vi "LED!!!!!s.vi"() -> ()   [LabVIEW 2020]
uses:
  LED GLOBALS!!!.vi
  LED-Global-string-length.vi
panel:
  out "Boolean":bool
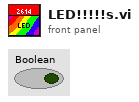
[diagram p1: front panel]
types:
  T1 = typedef "LED_Control_States.ctl" = enum16{"Config-Stripes", "swapperlines", "Rand", "Solid", "Flash-S", "Gradyent", "Move-Stripes", "Org-Rand", "Move-Point-Tail", "Flames", "Fade", "Alt-Colors"}
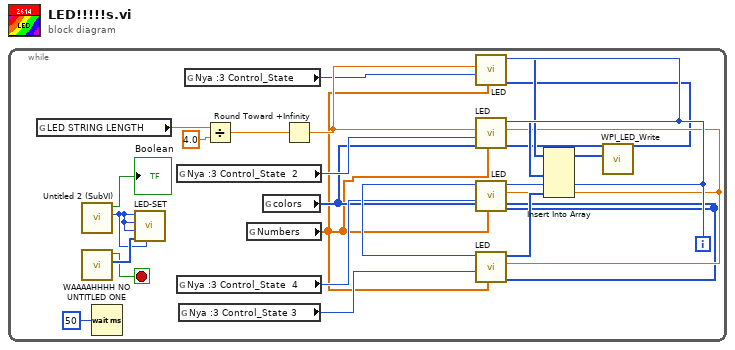
[diagram p0: block diagram]
diagram:
  n1 = while {
    i -> [w20]
    stop <- w3 stop-if-true
    n2 = global read "LED-Global-string-length.vi" "LED STRING LENGTH"() -> (w8:dbl)
    n3 = call "Untitled 2 (SubVI).vi"() -> ("Control_State"=w2:T1, "Boolean"=→"Boolean":bool)  [unwired: 10 in]
    n4 = call "WAAAAHHHH NO UNTITLED ONE.vi"() -> ("Array"=w4:u32[], "Boolean"=w3:bool)  [unwired: 10 in]
    n5 = Wait (ms)(milliseconds to wait=u32 50) -> ()  [unwired: 1 out]
    n6 = call "LED-SET.vi"("Control_State"=w2, "colors"=w4, "Control_State 2"=w2, "Control_State 3"=w2, "Control_State 4"=w2) -> ()  [unwired: 7 in]
    n7 = global read "LED GLOBALS!!!.vi" "Nya :3 Control_State  2"() -> (w11:T1)
    n8 = global read "LED GLOBALS!!!.vi" "Nya :3 Control_State  4"() -> (w9:T1)
    n9 = global read "LED GLOBALS!!!.vi" "Nya :3 Control_State 3"() -> (w10:T1)
    n10 = global read "LED GLOBALS!!!.vi" "Nya :3 Control_State"() -> (w12:T1)
    n11 = Divide(x=w8, y=4.0) -> (x/y=w15:dbl)
    n12 = global read "LED GLOBALS!!!.vi" "Numbers"() -> (w6:dbl[])
    n13 = global read "LED GLOBALS!!!.vi" "colors"() -> (w7:u32[])
    n14 = Round Toward +Infinity(x=w15) -> (ceil(x): smallest int >= x=w14:dbl)
    n15 = call "LED.vi"("Numbers"=w6, "colors"=w7, "Control_State"=w12, "Length"=w14, "Iteration_Num"=w20) -> ("Output_Array"=w19:u32[])  [unwired: 6 in]
    n16 = call "LED.vi"("Numbers"=w6, "colors"=w7, "Control_State"=w11, "Length"=w14, "Iteration_Num"=w20) -> ("Output_Array"=w18:u32[])  [unwired: 6 in]
    n17 = call "LED.vi"("Numbers"=w6, "colors"=w7, "Control_State"=w9, "Length"=w14, "Iteration_Num"=w20) -> ("Output_Array"=w17:u32[])  [unwired: 6 in]
    n18 = call "LED.vi"("Numbers"=w6, "colors"=w7, "Control_State"=w10, "Length"=w14, "Iteration_Num"=w20) -> ("Output_Array"=w16:u32[])  [unwired: 6 in]
    n19 = Insert Into Array(array=w19, new element #1=w18, new element #2=w17, new element #3=w16) -> (w13:u32[])  [unwired: 1 in]
    n20 = call <vilib>:"WPI_LED_Write.vi"("Color Array"=w13) -> ()  [unwired: 10 in, 1 out]
  }
